vi "Connect.vi"(4 "Error in":errorcluster, 5 "App state":T2, 6 "VISA resource name":refnum<visa-resource-name>, 7 "Semaphore":T1) -> (0 "Error out":errorcluster, 1 "App state":T2, 2 "VISA resource name":refnum<visa-resource-name>)   [LabVIEW 2020]
uses:
  Typedefs/State.ctl
  <vilib>/Instr/_visa.llb/VISA Configure Serial Port (Instr).vi
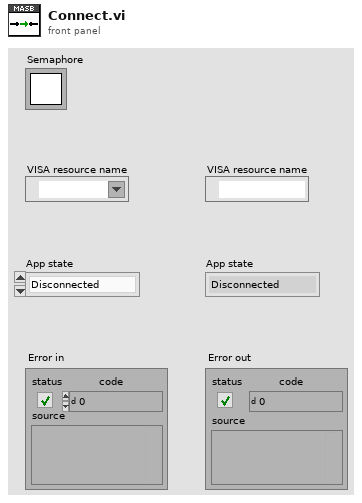
[diagram p1: front panel]
types:
  T1 = typedef "Semaphore RefNum" = refnum<k1>
  T2 = typedef "State.ctl" = enum16{"Disconnected", "Connected", "Measuring"}
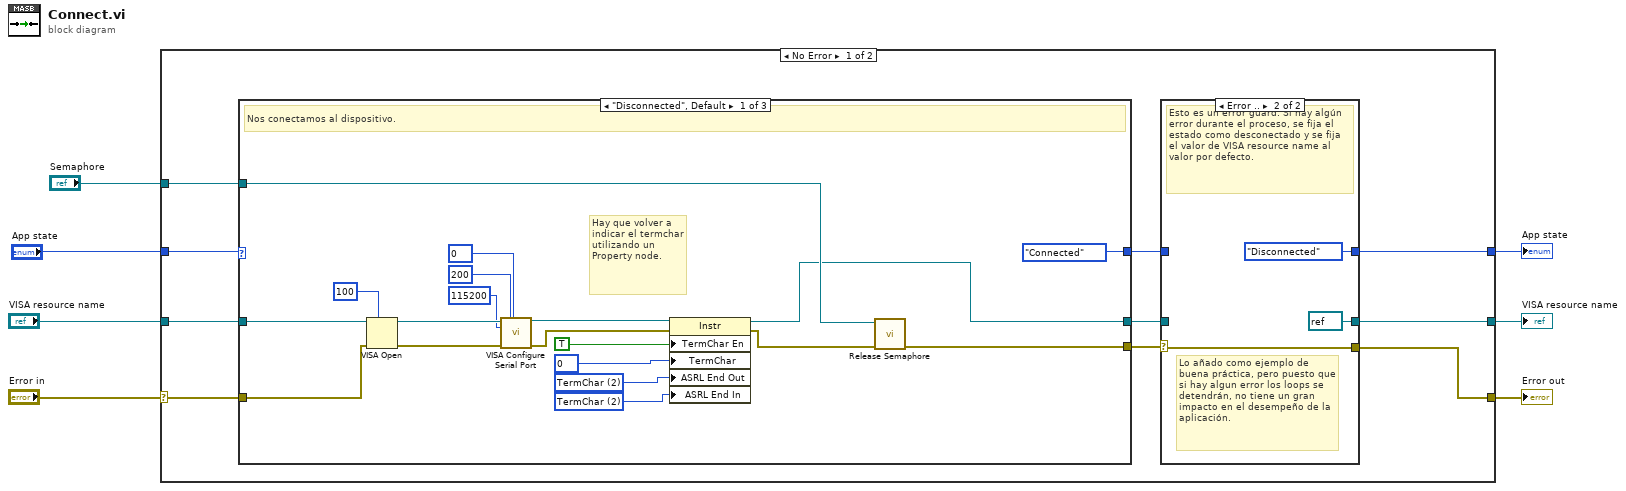
[diagram p0: block diagram]
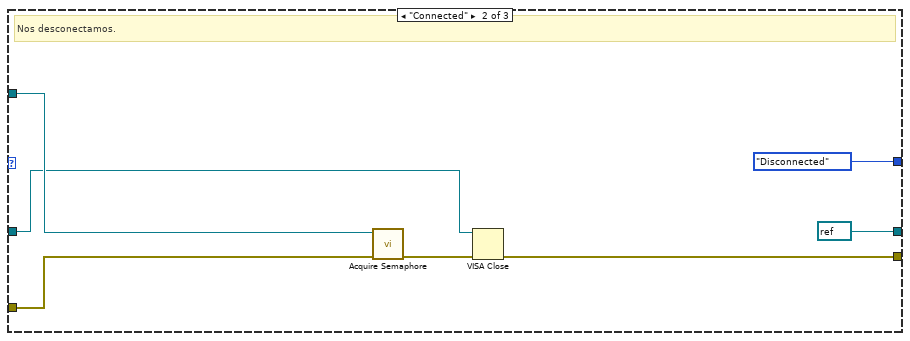
[diagram p2: hidden frame]
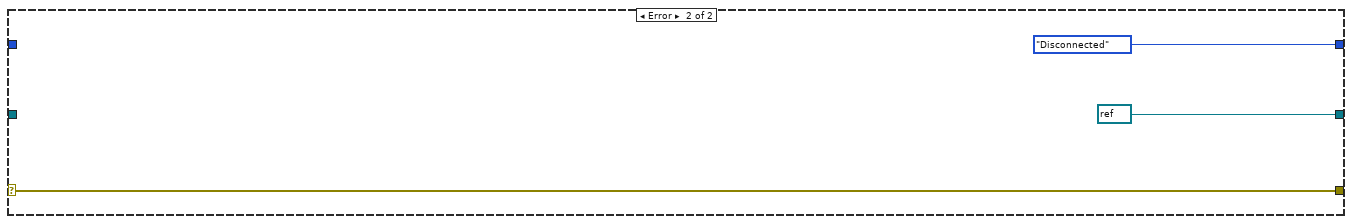
[diagram p5: hidden frame]
diagram:
  n1 = case shown="No Error" "Error in" {
    selector: "Error in" -> [w17 w53]
    tunnel: [w13 refnum<visa-resource-name> refnum ("VISA resource name out")] -> w6
    tunnel: "VISA resource name" -> [w16 _]
    tunnel: [w10 State."Disconnected" ("App state")] -> w4
    tunnel: [w12 w53] -> w3
    tunnel: "App state" -> [w9 _]
    tunnel: "Semaphore" -> [w8 _]
    frame No Error {
      n2 = case shown="\"Disconnected\", Default" w9 {
        selector: w9 -> [_ _ w46]
        tunnel: w17 -> [w24 w40 w44]
        tunnel: w16 -> [w23 w37 w45]
        tunnel: [w20 w43 w44] -> w15
        tunnel: [w18 refnum<visa-resource-name> refnum ("VISA resource name out") w45] -> w14
        tunnel: [State."Connected" ("App state") State."Disconnected" ("App state") w46] -> w11
        tunnel: w8 -> [w19 w38 _]
        frame "Disconnected", Default {
          w32 = u16 2 items=["None", "Last Bit", "TermChar"] ("Serial Settings:End Mode for Reads")
          w35 = u16 2 items=["None", "Last Bit", "TermChar", "Break"] ("Serial Settings:End Mode for Writes")
          # "Hay que volver a indicar el termchar utilizando un Property node."
          # "Nos conectamos al dispositivo."
          n3 = VISA Open(timeout (0)=u32 100 ("VISA Open timeout (0)"), error in (no error)=w24, VISA resource name=w23) -> (VISA resource name=w29:refnum<visa-resource-name>, error out=w31:errorcluster)  [unwired: 2 in]
          n4 = call-poly "VISA Configure Serial Port"("VISA resource name"=w29, "timeout (10sec)"=u32 200, "termination char\n(0xA = '\\n' = LF)"=u8 0 ("termination char\n(0xA = '\\n' = LF)"), "baud rate (9600)"=u32 115200, "error in (no error)"=w31) -> ("VISA resource name out"=w28:refnum<visa-resource-name>, "error out"=w30:errorcluster)  [unwired: 9 in]
          n5 = property class="Instr"(reference=w28, error in=w30, "TermChar En"=TRUE ("Message Based Settings:Termination Character Enable"), "TermChar"=u8 0 ("termination char\n(0xA = '\\n' = LF)"), "ASRL End Out"=w35, "ASRL End In"=w32) -> (reference out=w18:refnum<visa-resource-name>, error out=w21:errorcluster)
          n6 = call <vilib>:"Release Semaphore.vi"("error in (no error)"=w21, "semaphore"=w19) -> ("error out"=w20:errorcluster)  [unwired: 4 in, 1 out]
        }
        frame "Connected" {
          # "Nos desconectamos."
          n7 = call <vilib>:"Acquire Semaphore.vi"("error in (no error)"=w40, "semaphore"=w38) -> ("error out"=w39:errorcluster)  [unwired: 3 in, 2 out]
          n8 = VISA Close(VISA resource name=w37, error in (no error)=w39) -> (error out=w43:errorcluster)
        }
        frame "Measuring" {
        }
      }
      n9 = case shown="Error .." w15 {
        selector: w15 -> [w48 w50]
        tunnel: w14 -> [w49 _]
        tunnel: [w49 refnum<visa-resource-name> refnum ("VISA resource name out")] -> w13
        tunnel: [w47 State."Disconnected" ("App state")] -> w10
        tunnel: [w48 w50] -> w12
        tunnel: w11 -> [w47 _]
        frame No Error {
        }
        frame Error {
          # "Lo añado como ejemplo de buena práctica, pero puesto que si hay algun error los loops se detendrán, no tiene un gran impacto en el desempeño de la aplicación."
          # "Esto es un error guard. Si hay algún error durante el proceso, se fija el estado como desconectado y se fija el valor de VISA resource name al valor por defecto."
        }
      }
    }
    frame Error {
    }
  }
  "Error out" <- w3
  "VISA resource name" <- w6
  "App state" <- w4
